vi "svx_SC Line Autoscale.vi"(8 "State In":T1={"X Scale"={"Name"="Horizontal", "format string"="%#.2g", "Major Color"=16777238, "Minor Color"=16777216, "Scale Visible"=TRUE, " Label Visible"=TRUE, "Grid Style"=1, "Maximum"=1.0, "Minimum"=-1.0}, "Y Scale"={"Name"="Vertical", "format string"="%#.2g", "Major Color"=16777238, "Minor Color"=16777216, "Scale Visible"=TRUE, " Label Visible"=TRUE, "Grid Style"=1, "Maximum"=1.0, "Minimum"=-1.0}, "Plot"={"Point Style"=0, "Line Width"=0, "Line Style"=0, "Plot Color"=16860, "Point/fill"=16860}, "Arrow Color"=16860, "Autoscale"=TRUE, "Property Name"=[], "Container Bounds"={"Width"=550, "Height"=313}, "Background color"=16777226, "Annotation List"=[], "Cursor"={"Cursor Point Style"=13, "Cursor Style"=4, "Cursor Line Width"=1, "Cursor Line Style"=0, "Cursor Color"=16711680, "Cursor Name Visible"=TRUE, "Cursor Visible"=TRUE, "Cursor Position"={"X"=0.0, "Y"=0.0}, "Cursor Index"=0, "Lock Cursor Name"=FALSE, "Cursor reference"=0.0}, "size"=0, "Boundary Color"=9868950, "Maximum"=1.0, "Marker Point Style"=2, "Maker Visible"=TRUE, "Marker Color"=16860, "pair strings []"=[], "clearance boundary"=[{"boundary"={"x axis"=0.0, "y axis"=0.0}, "start point"=enum."center"}], "Custom pair name"=FALSE, "selector.visible"=TRUE, "Cursor Release"=refnum, "Children Tags"=[], "open?"=TRUE, "pair index"=[], "Legend Width"=200, " Parents Tags"="", "Label"="", "Legend Background"=16777226, "Legend Font"=16777222, "scale fit"=2, "user strings []"=[], "Item Width"=0, "out of state queue"=refnum, "property nodes"=refnum, "Kind"=enum."X-Scale", "Scale Range Change"=refnum} caption="State" {"pair index" min=0; "Y Scale"."Minimum" min=0.0; "Y Scale"."Maximum" min=0.0; "X Scale"."Minimum" min=0.0; "X Scale"."Maximum" min=0.0}, 11 "SC Line in":refnum<vi>) -> (0 "State Out":T1={"X Scale"={"Name"="Horizontal", "format string"="%#.2g", "Major Color"=16777238, "Minor Color"=16777216, "Scale Visible"=TRUE, " Label Visible"=TRUE, "Grid Style"=1, "Maximum"=1.0, "Minimum"=-1.0}, "Y Scale"={"Name"="Vertical", "format string"="%#.2g", "Major Color"=16777238, "Minor Color"=16777216, "Scale Visible"=TRUE, " Label Visible"=TRUE, "Grid Style"=1, "Maximum"=1.0, "Minimum"=-1.0}, "Plot"={"Point Style"=0, "Line Width"=0, "Line Style"=0, "Plot Color"=16860, "Point/fill"=16860}, "Arrow Color"=16860, "Autoscale"=TRUE, "Property Name"=[], "Container Bounds"={"Width"=550, "Height"=313}, "Background color"=16777226, "Annotation List"=[], "Cursor"={"Cursor Point Style"=13, "Cursor Style"=4, "Cursor Line Width"=1, "Cursor Line Style"=0, "Cursor Color"=16711680, "Cursor Name Visible"=TRUE, "Cursor Visible"=TRUE, "Cursor Position"={"X"=0.0, "Y"=0.0}, "Cursor Index"=0, "Lock Cursor Name"=FALSE, "Cursor reference"=0.0}, "size"=0, "Boundary Color"=9868950, "Maximum"=1.0, "Marker Point Style"=2, "Maker Visible"=TRUE, "Marker Color"=16860, "pair strings []"=[], "clearance boundary"=[{"boundary"={"x axis"=0.0, "y axis"=0.0}, "start point"=enum."center"}], "Custom pair name"=FALSE, "selector.visible"=TRUE, "Cursor Release"=refnum, "Children Tags"=[], "open?"=TRUE, "pair index"=[], "Legend Width"=200, " Parents Tags"="", "Label"="", "Legend Background"=16777226, "Legend Font"=16777222, "scale fit"=2, "user strings []"=[], "Item Width"=0, "out of state queue"=refnum, "property nodes"=refnum, "Kind"=enum."X-Scale", "Scale Range Change"=refnum} caption="State" {"pair index" min=0; "Y Scale"."Minimum" min=0.0; "Y Scale"."Maximum" min=0.0; "X Scale"."Minimum" min=0.0; "X Scale"."Maximum" min=0.0}, 1 "use queue?":bool, 3 "SC Line out":refnum<vi>)   [LabVIEW 2017, in "SVX SC Line.xctl"]
uses:
  <vilib>/addons/_XControls/Shaft Centerline/SVX SC Line.xctl
  <vilib>/addons/_XControls/Shaft Centerline/subVIs/svx_SC Line State.ctl
  <vilib>/addons/_XControls/Shaft Centerline/subVIs/svx_SC Line Bounds.ctl
  <vilib>/addons/_XControls/Shaft Centerline/subVIs/svx_SC Line Annotation List.ctl
  <vilib>/addons/_XControls/Shaft Centerline/subVIs/svx_SC Line OutState Queue.ctl
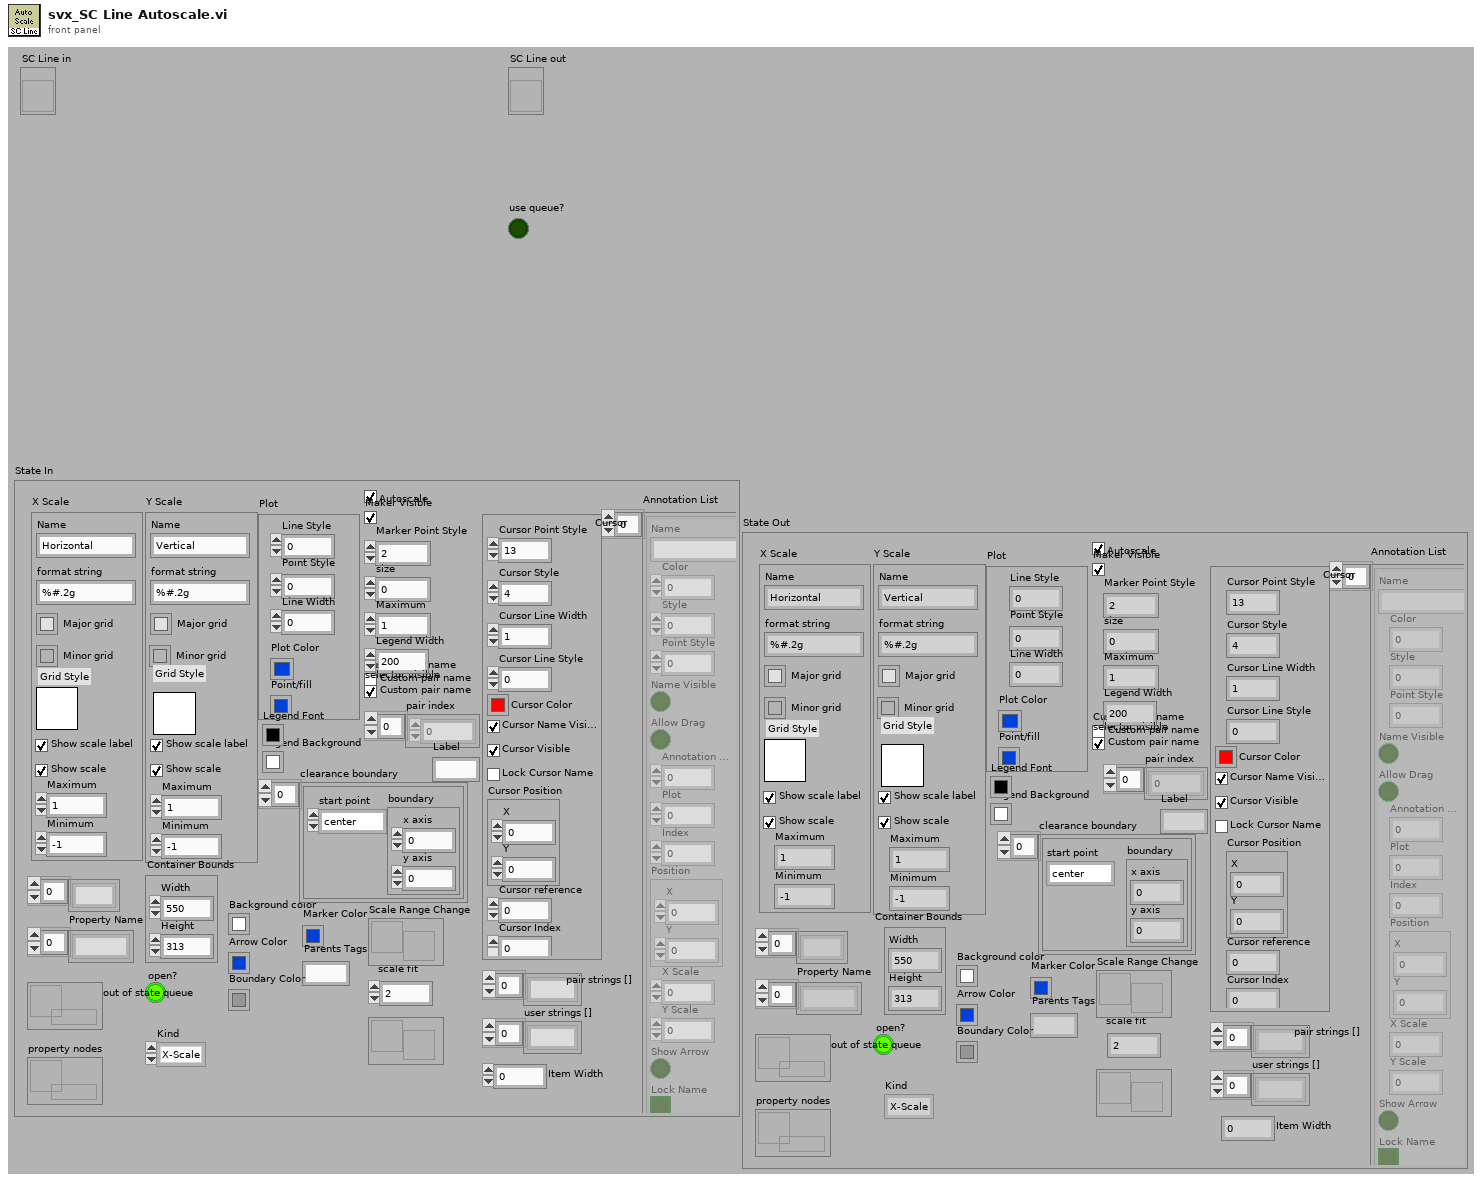
[diagram p1: front panel]
types:
  T1 = typedef "SVX SC Line.xctl/svx_SC Line State.ctl" = cluster{"X Scale":cluster{"Name":string, "format string":string, "Major Color":u32, "Minor Color":u32, "Scale Visible":bool, " Label Visible":bool, "Grid Style":u16, "Maximum":dbl, "Minimum":dbl}, "Y Scale":cluster{"Name":string, "format string":string, "Major Color":u32, "Minor Color":u32, "Scale Visible":bool, " Label Visible":bool, "Grid Style":u16, "Maximum":dbl, "Minimum":dbl}, "Plot":cluster{"Point Style":u8, "Line Width":u8, "Line Style":u8, "Plot Color":u32, "Point/fill":u32}, "Arrow Color":u32, "Autoscale":bool, "Property Name":string[], "Container Bounds":T2, "Background color":u32, "Annotation List":T3, "Cursor":cluster{"Cursor Point Style":u8, "Cursor Style":u8, "Cursor Line Width":u8, "Cursor Line Style":u8, "Cursor Color":u32, "Cursor Name Visible":bool, "Cursor Visible":bool, "Cursor Position":cluster{"X":dbl, "Y":dbl}, "Cursor Index":i32, "Lock Cursor Name":bool, "Cursor reference":dbl}, "size":i32, "Boundary Color":u32, "Maximum":dbl, "Marker Point Style":u8, "Maker Visible":bool, "Marker Color":u32, "pair strings []":string[], "clearance boundary":cluster{"boundary":cluster{"x axis":dbl, "y axis":dbl}, "start point":enum16{"center", "top", "bottom"}}[], "Custom pair name":bool, "selector.visible":bool, "Cursor Release":refnum<user-event>, "Children Tags":string[], "open?":bool, "pair index":i32[], "Legend Width":u32, " Parents Tags":string, "Label":string, "Legend Background":u32, "Legend Font":u32, "scale fit":u8, "user strings []":string[], "Item Width":u32, "out of state queue":T4, "property nodes":refnum<queue>, "Kind":enum16{"X-Scale", "Y-Scale", "Z-Scale"}, "Scale Range Change":refnum<user-event>}
  T2 = typedef "SVX SC Line.xctl/svx_SC Line Bounds.ctl" = cluster{"Width":u32, "Height":u32}
  T3 = typedef "SVX SC Line.xctl/svx_SC Line Annotation List.ctl" = cluster{"Name":string, "Color":u32, "Style":u8, "Point Style":u8, "Name Visible":bool, "Allow Drag":bool, "Annotation Mode":u32, "Plot":i32, "Index":i32, "Position":cluster{"X":dbl, "Y":dbl}, "X Scale":u32, "Y Scale":u32, "Show Arrow":bool, "Lock Name":bool, "Plot Area":i32, "Label Offset":cluster{"X":dbl, "Y":dbl}}[]
  T4 = typedef "SVX SC Line.xctl/svx_SC Line OutState Queue.ctl" = refnum<queue>
  T5 = cluster{"boundary":cluster{"x axis":dbl, "y axis":dbl}, "start point":enum16{"center", "top", "bottom"}}[]
  T6 = cluster{"orbit plot X":dbl[], "orbit plot Y":dbl[]}
  T7 = cluster{"boundary":cluster{"x axis":dbl, "y axis":dbl}, "start point":enum16{"center", "top", "bottom"}}
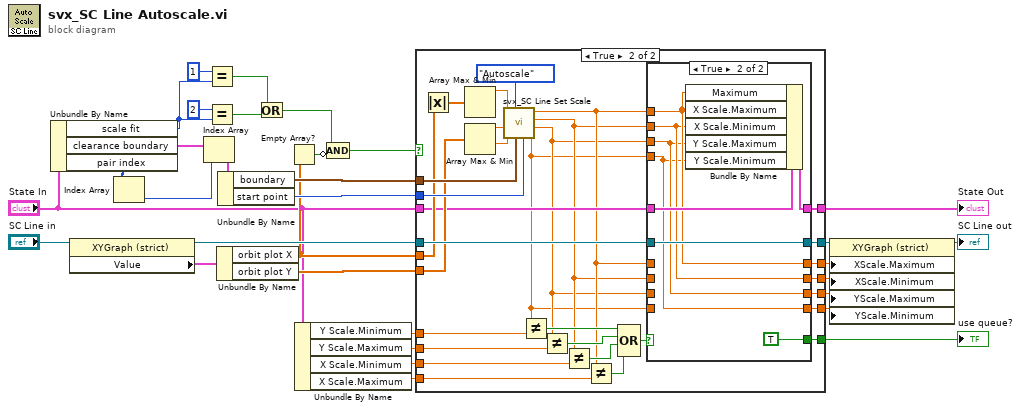
[diagram p0: block diagram]
diagram:
  n1 = Unbundle By Name("State In") -> ("scale fit"=w17:u8, "clearance boundary"=w31:T5, "pair index"=w20:i32[])
  n2 = property class="XYGraph (strict)"(reference="SC Line in") -> (reference out=w26:refnum<vi>, "Value"=w25:T6)  [unwired: 1 in, 1 out]
  n3 = Index Array(array=w20) -> (element=w19:i32)  [unwired: 1 in]
  n4 = Index Array(array=w31, index=w19) -> (element=w30:T7)
  n5 = Equal?(x=u8 1, y=w17) -> (x = y?=w14:bool)
  n6 = Equal?(x=u8 2, y=w17) -> (x = y?=w15:bool)
  n7 = Unbundle By Name(w25) -> ("orbit plot X"=w23:dbl[], "orbit plot Y"=w24:dbl[])
  n8 = Unbundle By Name(w30) -> ("boundary"=w29:cluster{"x axis":dbl, "y axis":dbl}, "start point"=w28:enum16{"center", "top", "bottom"})
  n9 = Or(x=w14, y=w15) -> (x .or. y?=w13:bool)
  n10 = Empty Array?(array=w23) -> (empty?=w22:bool)
  n11 = Unbundle By Name("State In") -> ("Y Scale.Minimum"=w11:dbl, "Y Scale.Maximum"=w10:dbl, "X Scale.Minimum"=w9:dbl, "X Scale.Maximum"=w8:dbl)
  n12 = Compound Arithmetic op=AND(w13, invert w22) -> (w21:bool)
  n13 = case shown="True" w21 {
    tunnel: [w38 w67] -> w7
    tunnel: w26 -> [w38 w68]
    tunnel: "State In" -> [w37 w57]
    tunnel: [w37 w63] -> w32
    tunnel: w29 -> [_ w61]
    tunnel: w28 -> [_ w60]
    tunnel: w23 -> [_ w59]
    tunnel: w24 -> [_ w58]
    tunnel: w11 -> [w33 w52]
    tunnel: w10 -> [w34 w51]
    tunnel: w9 -> [w35 w50]
    tunnel: w8 -> [w36 w49]
    tunnel: [w36 w48] -> w6
    tunnel: [w35 w47] -> w5
    tunnel: [w34 w46] -> w4
    tunnel: [w33 w45] -> w3
    tunnel: [_ w39] -> w2
    frame False {
    }
    frame True {
      n14 = Absolute Value(x=w59) -> (abs(x)=w69:dbl[])
      n15 = Array Max & Min(array=w69) -> (max value=w64:dbl)  [unwired: 3 out]
      n16 = Array Max & Min(array=w58) -> (max value=w66:dbl, min value=w65:dbl)  [unwired: 2 out]
      n17 = call <vilib>:"svx_SC Line Set Scale.vi"("start point"=w60, "boundary"=w61, "Selection"=enum16{"Autoscale", "X Scale", "Y Scale"}."Autoscale", "Y Min"=w65, "Y Max"=w66, "X Max"=w64) -> ("Y Minimum"=w41:dbl, "Y Maximum"=w42:dbl, "X Minimum"=w43:dbl, "X Maximum"=w44:dbl)  [unwired: 2 in]
      n18 = Not Equal?(x=w41, y=w52) -> (x != y?=w56:bool)
      n19 = Not Equal?(x=w42, y=w51) -> (x != y?=w55:bool)
      n20 = Not Equal?(x=w43, y=w50) -> (x != y?=w54:bool)
      n21 = Not Equal?(x=w44, y=w49) -> (x != y?=w53:bool)
      n22 = Compound Arithmetic op=OR(w56, w55, w54, w53) -> (w40:bool)
      n23 = case shown="True" w40 {
        tunnel: w68 -> [w74 w81]
        tunnel: [w74 w81] -> w67
        tunnel: [w75 w83] -> w63
        tunnel: w57 -> [w75 w82]
        tunnel: w41 -> [_ w77]
        tunnel: w42 -> [_ w78]
        tunnel: w43 -> [_ w79]
        tunnel: w44 -> [_ w80]
        tunnel: [w73 w80] -> w48
        tunnel: [w72 w79] -> w47
        tunnel: [w71 w78] -> w46
        tunnel: [w70 w77] -> w45
        tunnel: w44 -> [w73 _]
        tunnel: w43 -> [w72 _]
        tunnel: w42 -> [w71 _]
        tunnel: w41 -> [w70 _]
        tunnel: [_ TRUE ("use queue?")] -> w39
        frame False {
        }
        frame True {
          n24 = Bundle By Name(cluster=w82, "Maximum"=w80, "X Scale.Maximum"=w80, "X Scale.Minimum"=w79, "Y Scale.Maximum"=w78, "Y Scale.Minimum"=w77) -> (w83:T1)
        }
      }
    }
  }
  "State Out" <- w32
  "use queue?" <- w2
  n25 = property class="XYGraph (strict)"(reference=w7, "XScale.Maximum"=w6, "XScale.Minimum"=w5, "YScale.Maximum"=w4, "YScale.Minimum"=w3) -> (reference out=→"SC Line out":refnum<vi>)  [unwired: 1 in, 1 out]
